vi "main.vi"() -> ()   [LabVIEW 2014]
uses:
  typedef/ctlPlot.ctl
  typedef/ePMUConfig.ctl
  typedef/eStepType.ctl
  typedef/eStepDir.ctl
  typedef/rdoTestType.ctl
  typedef/appState.ctl
  typedef/eRptType.ctl
  typedef/PMUConfig.ctl
panel:
  out "Uncertainties":dbl[][][](array[numeric]) format="%#_2g"
  in  "rdoTest Type":T1
  in  "btnSave":bool
  in  "btnCalcPFI":bool
  in  "btnCalcRT":bool
  in  "DONE":bool
  in  "Tab Control":T2(tab)
  in  "UncertPage":enum16{"50 Hz", "60 Hz"}(ring) caption="Nominal Freq"
  out "Uncert Table":string[][](table)
  out "StepLimits":dbl[][][](array[numeric]) caption="Step Test Limits" format="%#_4f"
  in  "Limit Page":T3 caption="PMU Config"
  out "Limits":dbl[][][](array[numeric]) caption="TVE, FE, RFE Limits"
  in  "btnSaveTUR":bool
  out "TUR":dbl[][][](array[numeric])
  in  "TUR Page":T3 caption="PMU Config"
  in  "full_temp_PFI":enum32{"full", "temp"}(tab)
  in  "PFI Page":T3 caption="PMU Config"
  out "PFI":string[][][](array[string])
  out "Temp Test PFI":string[][][](array[string])
  in  "TempFreq":enum16{"50 Hz", "60 Hz"}(ring) caption="Nominal Freq"
  out "RTPFI":string[][][](array[string]) caption="Pass/Fail/Indeterminate"
  in  "eRTDir":T4 caption="Step Direction"
  in  "eRTType":T5 caption="Step Type"
  out "RTUncert":dbl[][][][][](array[numeric]) caption="Resp Time Uncert"
  out "RTRange":dbl[][][][][](array[numeric]) caption="Resp Time Range"
  in  "eRTPage":T3 caption="PMU Config"
  out "DlyTimePFI":string[][][](array[string])
  in  "eDTDir":T4 caption="Step Direction"
  in  "eDTType":T5 caption="Step Type"
  in  "eDTPage":T3 caption="PMU Config"
  out "DlyTimeRng":dbl[][][][][](array[numeric]) format="%.6f"
  in  "eOvrDir":T4 caption="Step Direction"
  in  "eOvrType":T5 caption="Step Type"
  in  "eOvrUndrPage":T3 caption="PMU Config"
  out "OvrUndrPFI":string[][][][][](array[string])
  out "OvrUndr":dbl[][][][][](array[numeric])=[[[[[5.598492295160192, 5.589160017980474, 5.579827740800756, 6.2090278478135055, 6.202935187769419, 6.196842527725332, 6.270368754436869, 6.261733208094874, 6.2530976617528795, 5.499241138114173, 5.4912209769255735, 5.483200815736974, 5.591363005137677, 5.589161707344972, 5.586960409552266, 6.2034021327898525, 6.2029551231392706, 6.202508113488689, 6.262186470202315, 6.261747037530138, 6.261307604857961, 5.492149609028501, 5.491120362323346, 5.490091115618191], [4.582281382800085, 4.572949105620367, 4.563616828440649, 2.0737377226338936, 2.0676450625898064, 2.0615524025457193, 1.1136472889469742, 1.1050117426049793, 1.0963761962629843, 4.500837324127726, 4.492817162939127, 4.484797001750527, 4.57515178562041, 4.572950487827704, 4.570749190034999, 2.068098717363672, 2.06765170771309, 2.067204698062508, 1.1054536157657309, 1.1050141830935536, 1.1045747504213763, 4.493764088606066, 4.492734841900911, 4.491705595195756], [6.26023399342542, 6.250901716245702, 6.241569439065984, 6.128438171518977, 6.12234551147489, 6.116252851430803, 6.430675694174775, 6.422040147832781, 6.413404601490786, 6.102855597590311, 6.094835436401712, 6.086815275213112, 6.253149166340811, 6.2509478685481055, 6.2487465707554, 6.122858708702316, 6.122411699051734, 6.121964689401152, 6.422526817417168, 6.422087384744991, 6.421647952072814, 6.095816462969536, 6.094787216264381, 6.093757969559226], [3.375202432081235, 3.3658701549015175, 3.3565378777218, 3.302740243145951, 3.296647583101864, 3.2905549230577766, 1.1419367489007164, 1.1333012025587215, 1.1246656562167265, 2.0396319733224955, 2.0316118121338955, 2.0235916509452956, 3.368096303933992, 3.3658950061412862, 3.3636937083485803, 3.297130232216894, 3.296683222566312, 3.29623621291573, 1.1337489711565862, 1.133309538484409, 1.1328701058122317, 2.0326249854599556, 2.0315957387548007, 2.030566492049646]], [[5.6114389386325305, 5.602495822485004, 5.593552706337477, 6.4971644746473425, 6.4906779148884395, 6.4841913551295365, 6.452789687138199, 6.442635198982573, 6.432480710826947, 5.499700075652654, 5.491172020965302, 5.4826439662779505, 5.604365790119637, 5.602470106718821, 5.600574423318005, 6.491501742716185, 6.490751963178685, 6.4900021836411845, 6.443115798655941, 6.442548550239463, 6.4419813018229855, 5.492187667629821, 5.4911167638448894, 5.490045860059958], [4.592803334544344, 4.583860218396818, 4.574917102249291, 1.1519003094451032, 1.1454137496861998, 1.1389271899272964, 2.1576995544831505, 2.147545066327524, 2.1373905781718974, 4.501305162749851, 4.4927771080625, 4.484249053375148, 4.585734861625306, 4.58383917822449, 4.5819434948236735, 1.146176596569033, 1.1454268170315325, 1.144677037494032, 2.148083431829625, 2.1475161834131473, 2.1469489349966695, 4.4938028014762015, 4.49273189769127, 4.491660993906338], [5.824200079831354, 5.815256963683828, 5.806313847536301, 6.213851725577966, 6.207365165819063, 6.20087860606016, 6.175131282852548, 6.164976794696922, 6.154822306541296, 6.103387438698514, 6.094859384011162, 6.08633132932381, 5.81714404673894, 5.815248363338124, 5.813352679937307, 6.208174990295637, 6.207425210758137, 6.206675431220637, 6.165428416601619, 6.1648611681851415, 6.164293919768664, 6.095893577165425, 6.094822673380493, 6.093751769595562], [3.140235327361881, 3.1312922112143546, 3.1223490950668285, 1.101903941962272, 1.0954173822033686, 1.0889308224444652, 2.0651467530546004, 2.054992264898974, 2.044837776743347, 2.040147849357748, 2.0316197946703958, 2.0230917399830437, 3.133183263659809, 3.131287580258993, 3.1293918968581766, 1.0961777579065755, 1.095427978369075, 1.0946781988315746, 2.0555209711448583, 2.0549537227283805, 2.0543864743119027, 2.032678461578429, 2.0316075577934978, 2.0305366540085665]]]]] caption="Overshoot in Percent (%)" format="%.2f"
  out "StepPlot":cluster{"Array":dbl[], "Array":dbl[]}(graph)
  in  "ctlPlot":T6
  out "Step TVE":cluster{"Array":dbl[], "Array":dbl[]}(graph)
  in  "ePlotPage":T3 caption="PMU Config"
  in  "ePlotType":enum16{"Phase", "Magnitude"}(ring) caption="Step Type"
  in  "ePlotDir":enum16{"Pos", "Neg"}(ring) caption="Step Direction"
  out "error out":errorcluster
  in  "error in (no error)":errorcluster
  # "VC"
  # "IA"
  # "VB"
  # "V+"
  # "IB"
  # "IC"
  # "I+"
  # "FREQ"
  # "ROCOF"
  # "VA"
  # "Step Resp Time (s)"
  # "Step Delay Time (s)"
  # "Step Ovr/Undr  (%)"
  # "VA TVE"
  # "VB TVE"
  # "VC TVE"
  # "V+ TVE"
  # "IA TVE"
  # "IB TVE"
  # "IC TVE"
  # "I+ TVE"
  # "FE"
  # "RFE"
  # "FreqRng"
  # "MagRng"
  # "Harm"
  # "OOB"
  # "Phase Mod"
  # "Ampl Mod"
  # "Ramp +"
  # "Ramp -"
  # "VA"
  # "VB"
  # "VC"
  # "V+"
  # "IA"
  # "IB"
  # "IC"
  # "I+"
  # "FREQ"
  # "ROCOF"
  # "FreqRng"
  # "MagRng"
  # "Harm"
  # "OOB"
  # "Phase Mod"
  # "Ampl Mod"
  # "Ramp +"
  # "Ramp -"
  # "VA TVE"
  # "VB TVE"
  # "VC TVE"
  # "V+ TVE"
  # "IA TVE"
  # "IB TVE"
  # "IC TVE"
  # "I+ TVE"
  # "FE"
  # "RFE"
  # "FreqRng"
  # "MagRng"
  # "Harm"
  # "OOB"
  # "Phase Mod"
  # "Ampl Mod"
  # "Freq Ramp +"
  # "Freq Ramp -"
  # "60F0_10Fs_M_50C\n\n60F0_10Fs_M_50C\n\n60F0_10Fs_P_50C\n\n60F0_10Fs_P_0C\n\n60F0_12Fs_M_50C\n\n60F0_12Fs_M_0C\n\n60F0_12Fs_P_50C\n\n60F0_12Fs_P_0C\n\n60F0_15Fs_M_50C\n\n60F0_15Fs_M_0C\n\n60F0_15Fs_P_50C\n\n60F0_15Fs_P_0C\n\n60F0_20Fs_M_50C\n\n60F0_20Fs_M_0C\n\n60F0_20Fs_P_50C\n\n60F0_20Fs_P_0C\n\n60F0_30Fs_M_50C\n\n60F0_30Fs_M_0C\n60F0_30Fs_P_50C\n\n60F0_30Fs_P_0C\n\n60F0_60Fs_M_50C\n\n60F0_60Fs_M_0C\n\n60F0_60Fs_P_50C\n\n60F0_60Fs_P_0C"
  # "50F0_10Fs_M_50C\n\n50F0_10Fs_M_0C\n\n50F0_10F0_P_50C\n\n50F0_10Fs_P_0C\n\n50F0_25Fs_M_50C\n\n50F0_25Fs_M_0C\n\n50F0_25Fs_P_50C\n\n50F0_25Fs_P_0C\n\n50F0_50Fs_M_50C\n\n50F0_50Fs_M_0C\n\n50F0_50Fs_P_50C\n\n50F0_50Fs_P_0C"
  # "VA TVE"
  # "VB TVE"
  # "VC TVE"
  # "V+ TVE"
  # "IA TVE"
  # "IB TVE"
  # "IC TVE"
  # "I+ TVE"
  # "FE"
  # "RFE"
  # "VA                      VB                     VC                     V+                     IA                         IB                    IC                            I+                  Freq                    ROCOF"
  # "Phase Step Positive RT"
  # "Phase Step Negative RT"
  # "Magnitude Step Positive RT"
  # "Magnitude Step Positive RT"
  # "VA                      VB                     VC                     V+                     IA                         IB                    IC                            I+                  Freq                    ROCOF"
  # "plus\n\nRT\n\nminus"
  # "VA                      VB                     VC                     V+                     IA                         IB                    IC                            I+                  Freq                    ROCOF"
  # "RT + unc\n\nRT\n\nRT - unc"
  # "VA"
  # "VB"
  # "VC"
  # "V+"
  # "IA"
  # "IB"
  # "IC"
  # "I+"
  # "Phase Step Pos"
  # "Phase Step Neg"
  # "Mag Step Pos"
  # "Mag Step Neg"
  # "VA"
  # "VB"
  # "VC"
  # "V+"
  # "IA"
  # "IB"
  # "IC"
  # "I+"
  # "DT + Unc"
  # "DT"
  # "DT - Unc"
  # "VA"
  # "VB"
  # "VC"
  # "V+"
  # "IA"
  # "IB"
  # "IC"
  # "I+"
  # "PreOvr"
  # "PreUndr"
  # "PostOvr"
  # "PostUndr"
  # "VA+u"
  # "VA"
  # "VA-u"
  # "VB+u"
  # "VB"
  # "VB-u"
  # "VC+u"
  # "VCB"
  # "VC-u"
  # "V+u"
  # "V+B"
  # "V+-u"
  # "IA+u"
  # "IA"
  # "IA-u"
  # "IB+u"
  # "IB"
  # "IB-u"
  # "IC+u"
  # "IC"
  # "IC-u"
  # "I++u"
  # "I+B"
  # "I+-u"
  # "PreOvr"
  # "PreUndr"
  # "PostOvr"
  # "PostUndr"
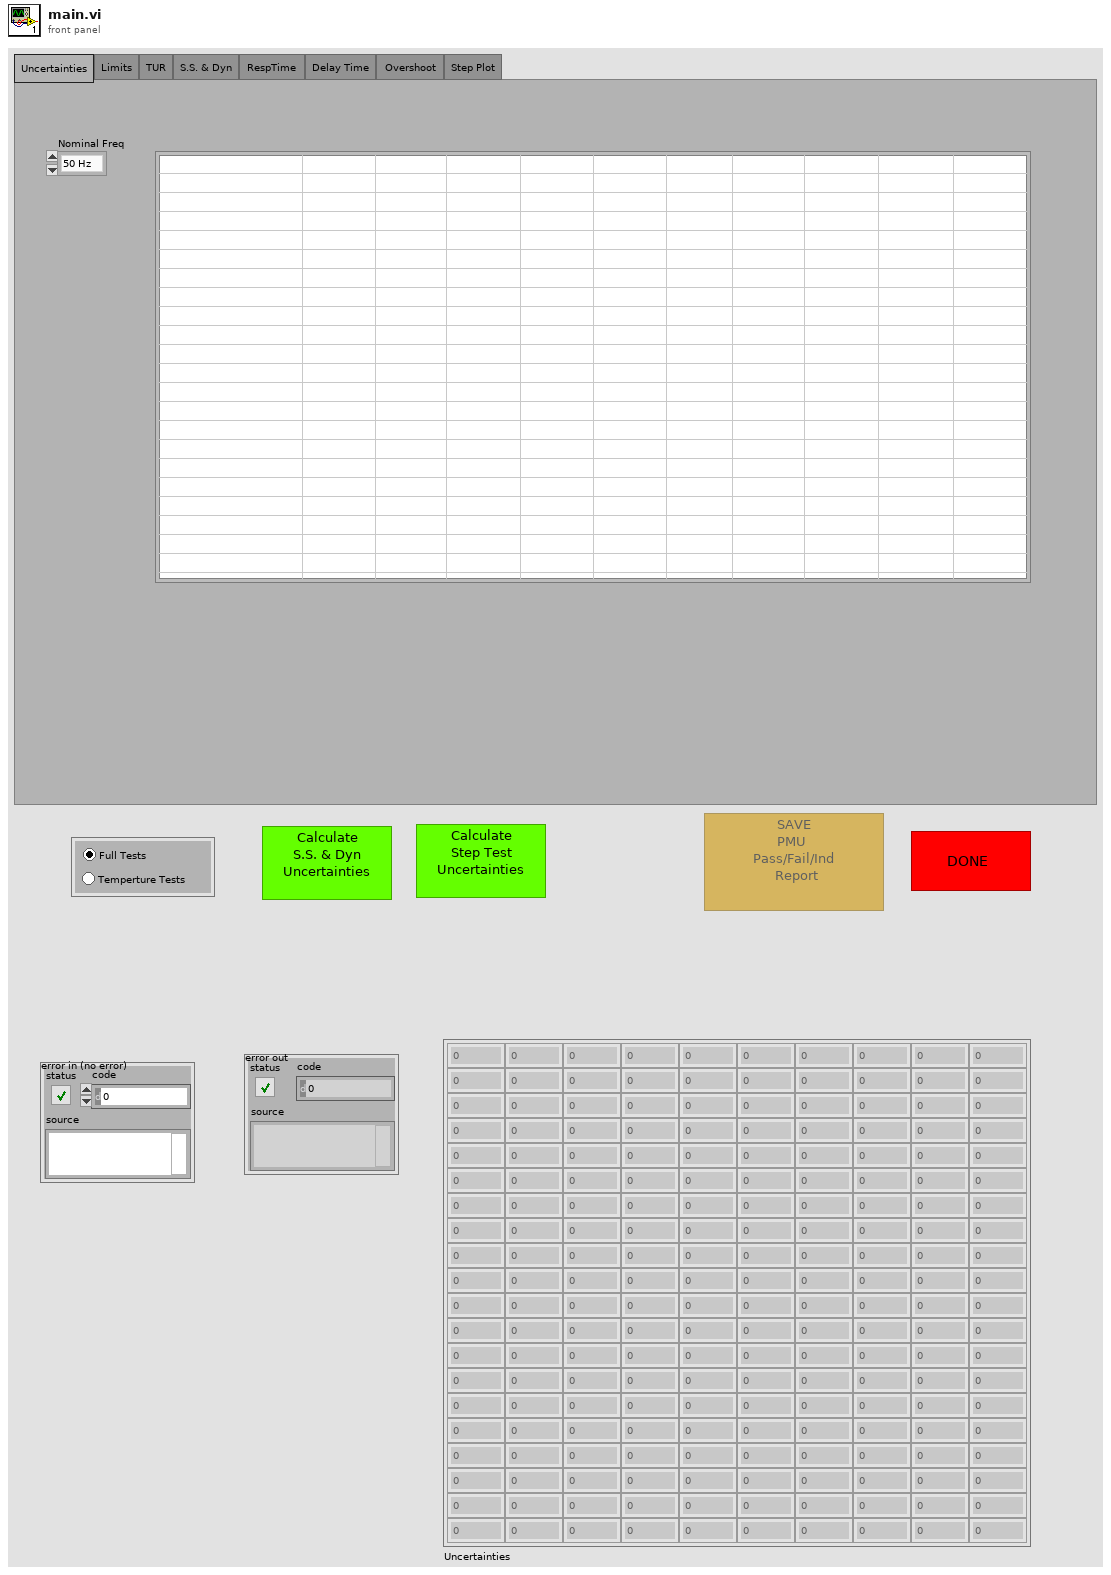
[diagram p1: front panel]
types:
  T1 = typedef "rdoTestType.ctl" = enum32{"rFull", "rTemp"}
  T2 = enum32{"Uncertainties", "Limits", "TUR", "S.S. & Dyn", "RespTime ", "Delay Time", "Overshoot ", "Step Plot"}
  T3 = typedef "ePMUConfig.ctl" = enum16{"50F0 10Fs M", "50F0 10Fs P", "50F0 25Fs M", "50F0 25Fs P", "50F0 50Fs M", "50F0 50Fs P", "60F0 10Fs M", "60F0 10Fs P", "60F0 12Fs M", "60F0 12Fs P", "60F0 15Fs M", "60F0 15Fs P", "60F0 20Fs M", "60F0 20Fs P", "60F0 30Fs M", "60F0 30Fs P", "60F0 60Fs M", "60F0 60Fs P"}
  T4 = typedef "eStepDir.ctl" = enum16{"Pos", "Neg"}
  T5 = typedef "eStepType.ctl" = enum16{"Phase", "Magnitude"}
  T6 = typedef "ctlPlot.ctl" = cluster{"Channel":enum16{"VA", "VB", "VC", "V+", "IA", "IB", "IC", "I+", "FREQ", "ROCOF"}, "Parameter":enum16{"TVE", "ME", "PE"}}
  T7 = enum8{"Enabled", "Disabled", "Disabled and Grayed Out"}
  T8 = typedef "appState.ctl" = enum16{"init", "processUI", "exit"}
  T9 = typedef "eRptType.ctl" = enum16{"get", "Clear", "Set Temp", "Set PFI", "Set Step"}
  T10 = typedef "PMUConfig.ctl" = cluster{"Class":string, "Fs":dbl, "F0":dbl}
  T11 = enum16{"get", "Clear", "Set Temp", "Set PFI", "Set Step"}
  T12 = cluster{"DlyTimeRng":dbl[][][][][], "DlyTimePFI":string[][][]}
  T13 = cluster{"OvrUndr":dbl[][][][][], "OvrUndrPFI":string[][][][][]}
  T14 = cluster{"RT Range":dbl[][][][][], "RT Uncert":dbl[][][][][], "RT_PFI":string[][][]}
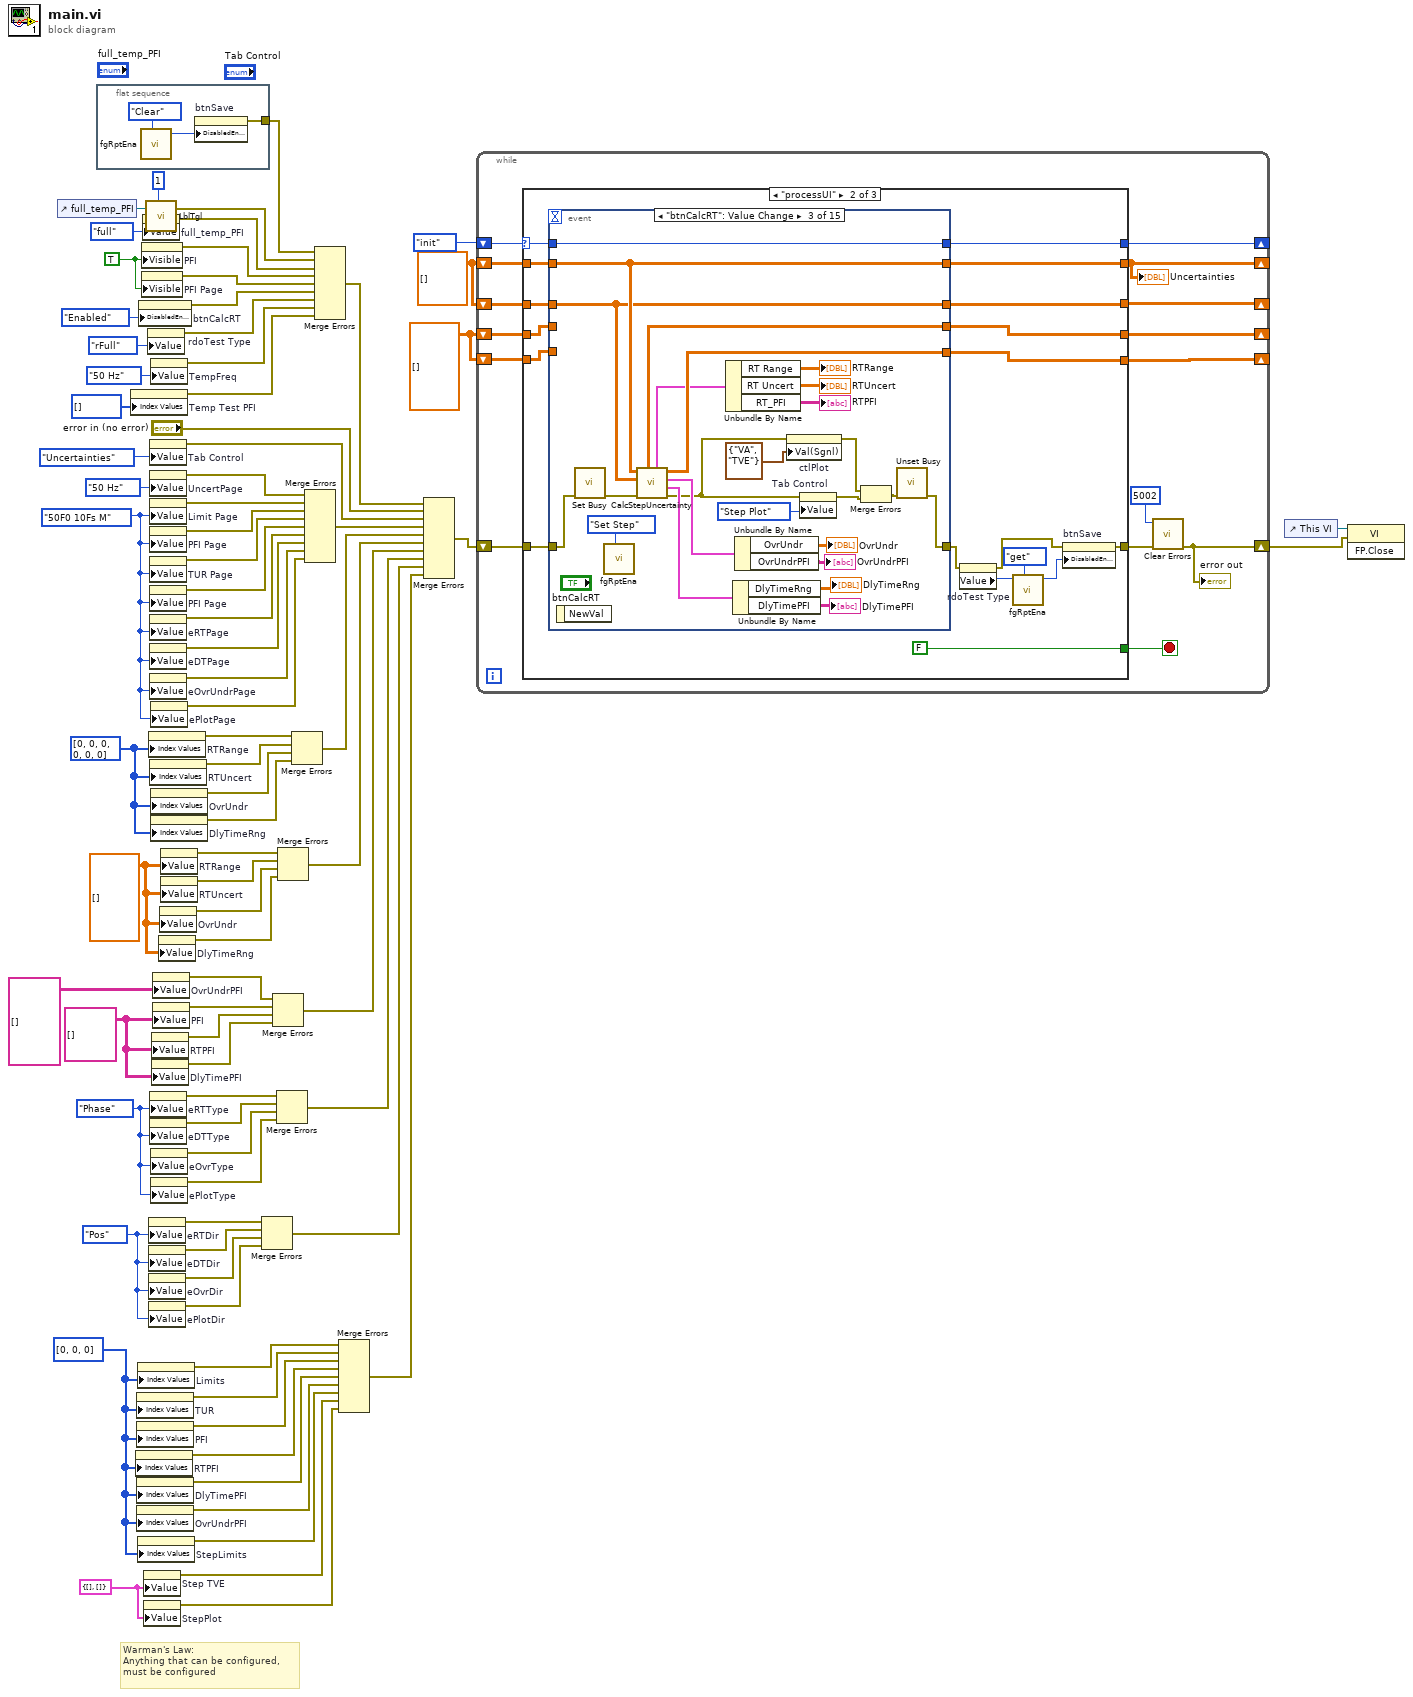
[diagram p0: block diagram]
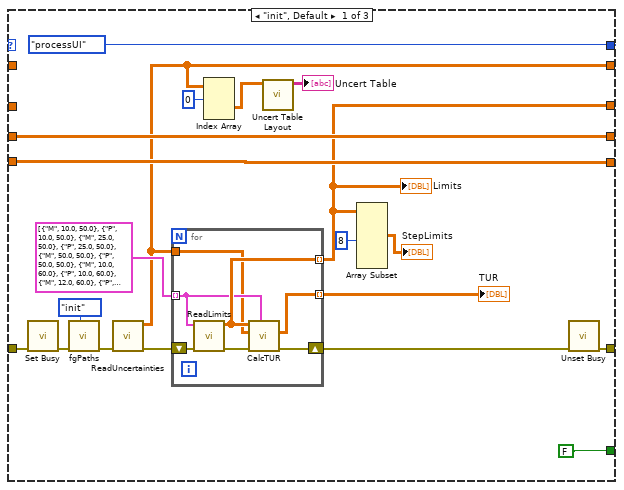
[diagram p2: hidden frame]
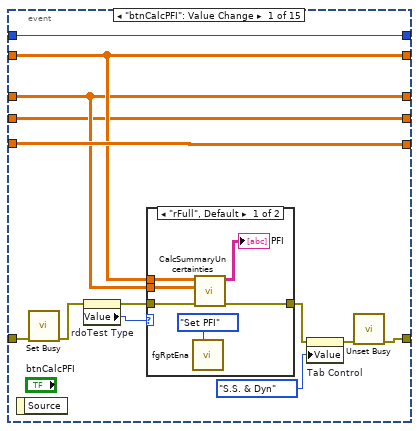
[diagram p3: hidden frame]
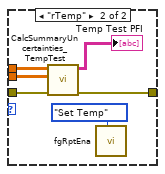
[diagram p4: hidden frame]
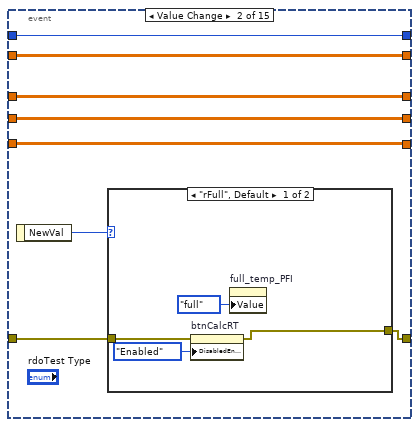
[diagram p5: hidden frame]
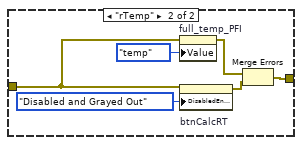
[diagram p6: hidden frame]
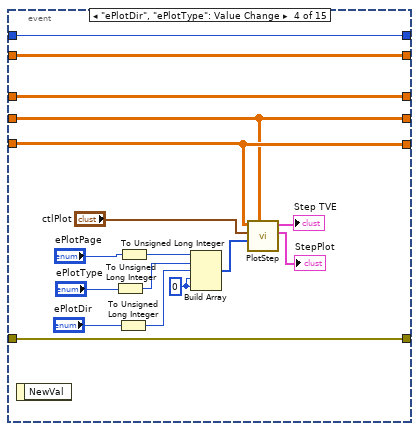
[diagram p7: hidden frame]
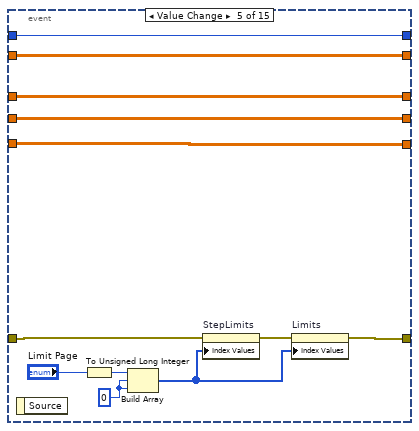
[diagram p8: hidden frame]
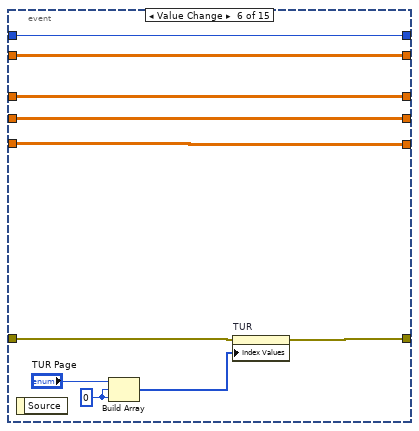
[diagram p9: hidden frame]
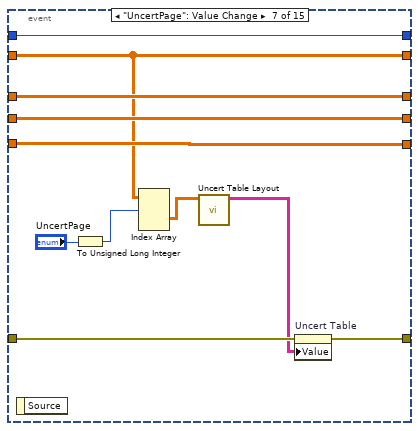
[diagram p10: hidden frame]
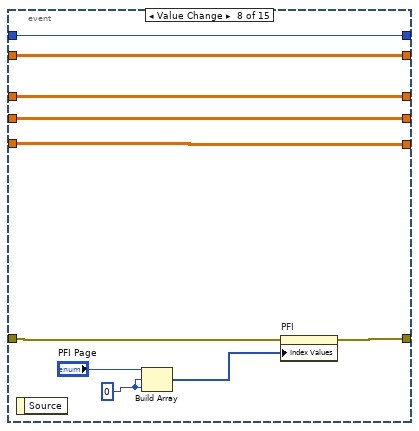
[diagram p11: hidden frame]
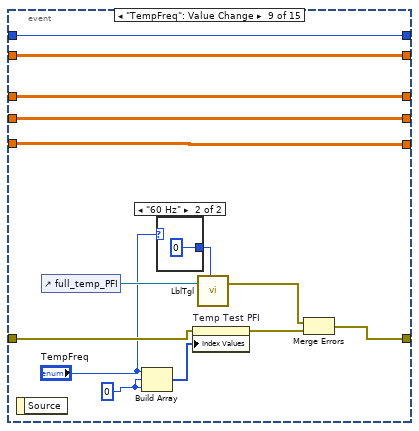
[diagram p12: hidden frame]
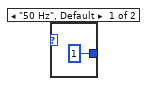
[diagram p13: hidden frame]
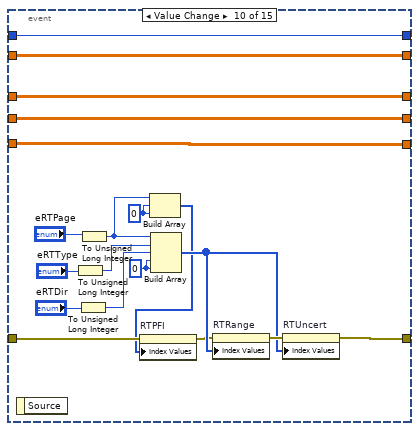
[diagram p14: hidden frame]
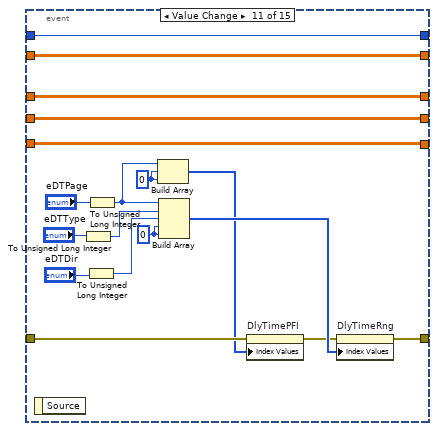
[diagram p15: hidden frame]
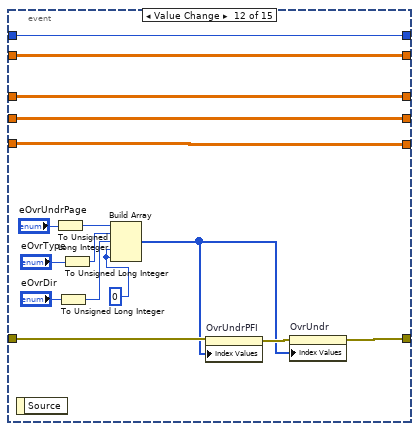
[diagram p16: hidden frame]
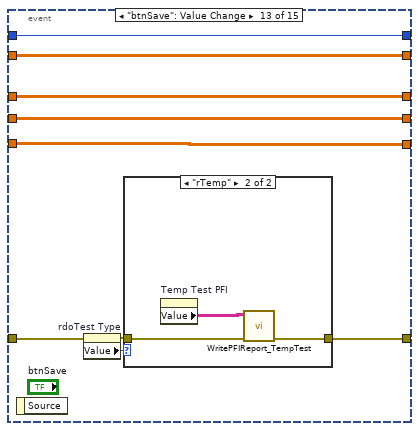
[diagram p17: hidden frame]
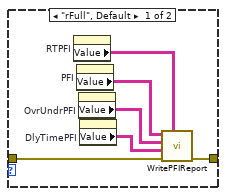
[diagram p18: hidden frame]
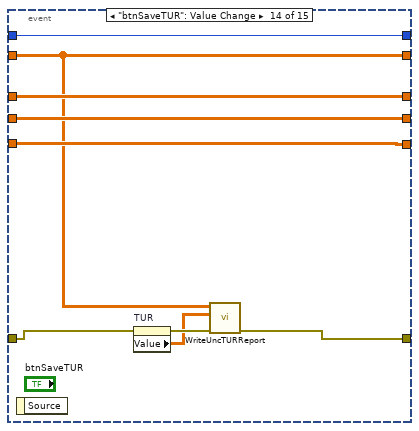
[diagram p19: hidden frame]
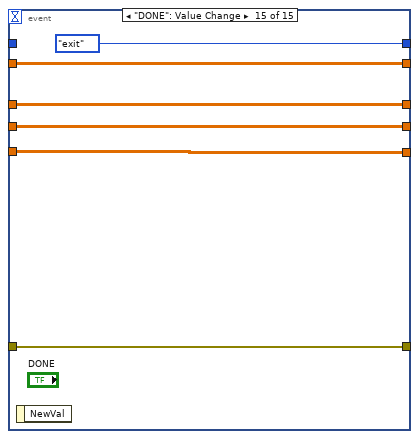
[diagram p20: hidden frame]
diagram:
  w10 = TRUE ("Visible")
  w21 = cluster{"Array":dbl[], "Array":dbl[]} {"Array"=[], "Array"=[]} ("Step TVE")
  w43 = eStepDir."Pos" ("eRTDir")
  w48 = eStepType."Phase" ("eRTType")
  w59 = u32[] [0, 0, 0, 0, 0, 0] ("Index Values")
  w30 = string[][][] [] ("PFI")
  w71 = dbl[][][][][] [] ("Range")
  w50 = ePMUConfig."50F0 10Fs M" ("Limit Page")
  w23 = u32[] [0, 0, 0] ("Index Values")
  w74 = dbl[][][][][] [] ("Step Data")
  w78 = dbl[][][] []
  # "Warman's Law:\nAnything that can be configured,\nmust be configured"
  n1 = control-ref of="full_temp_PFI"() -> (w82:refnum<vi>)
  n2 = flat-sequence {
    tunnel: [w84] -> w2
    frame #0 {
      n3 = call "fgRptEna.vi"("eRptType"=eRptType."Clear" ("Enum")) -> ("ENA"=w83:T7)  [unwired: 10 in]
      n4 = property on="btnSave" class="Bool"("DisabledEnum"=w83) -> (error out=w84:errorcluster)  [unwired: 2 in, 1 out]
    }
  }
  n5 = property on="Temp Test PFI" class="Arr (strict)"("Index Values"=u32[] []) -> (error out=w3:errorcluster)  [unwired: 2 in, 1 out]
  n6 = property on="RTPFI" class="Arr (strict)"("Index Values"=w23) -> (error out=w66:errorcluster)  [unwired: 2 in, 1 out]
  n7 = property on="TUR" class="Arr (strict)"("Index Values"=w23) -> (error out=w68:errorcluster)  [unwired: 2 in, 1 out]
  n8 = property on="PFI" class="Arr (strict)"("Index Values"=w23) -> (error out=w67:errorcluster)  [unwired: 2 in, 1 out]
  n9 = property on="DlyTimePFI" class="Arr (strict)"("Index Values"=w23) -> (error out=w65:errorcluster)  [unwired: 2 in, 1 out]
  n10 = property on="OvrUndrPFI" class="Arr (strict)"("Index Values"=w23) -> (error out=w64:errorcluster)  [unwired: 2 in, 1 out]
  n11 = property on="Limits" class="Arr (strict)"("Index Values"=w23) -> (error out=w69:errorcluster)  [unwired: 2 in, 1 out]
  n12 = property on="StepLimits" class="Arr (strict)"("Index Values"=w23) -> (error out=w22:errorcluster)  [unwired: 2 in, 1 out]
  n13 = property on="btnCalcRT" class="Bool"("DisabledEnum"=T7."Enabled" ("Disabled")) -> (error out=w12:errorcluster)  [unwired: 2 in, 1 out]
  n14 = property on="PFI" class="Arr (strict)"("Visible"=w10) -> (error out=w14:errorcluster)  [unwired: 2 in, 1 out]
  n15 = property on="PFI Page" class="Enum (strict)"("Visible"=w10) -> (error out=w15:errorcluster)  [unwired: 2 in, 1 out]
  n16 = property on="full_temp_PFI" class="TabCtl (strict)"("Value"=enum32{"full", "temp"}."full" ("full_temp_PFI")) -> (error out=w8:errorcluster)  [unwired: 2 in, 1 out]
  n17 = property on="Step TVE" class="XYGraph (strict)"("Value"=w21) -> (error out=w20:errorcluster)  [unwired: 2 in, 1 out]
  n18 = property on="StepPlot" class="XYGraph (strict)"("Value"=w21) -> (error out=w19:errorcluster)  [unwired: 2 in, 1 out]
  n19 = call "LblTgl.vi"("TabControl in"=w82, "Numeric"=1) -> ("error out"=w7:errorcluster)  [unwired: 17 in]
  n20 = property on="rdoTest Type" class="RadioBtnsControl (strict)"("Value"=enum32{"rFull", "rTemp"}."rFull" ("Test Type")) -> (error out=w11:errorcluster)  [unwired: 2 in, 1 out]
  n21 = property on="RTRange" class="Arr (strict)"("Index Values"=w59) -> (error out=w63:errorcluster)  [unwired: 2 in, 1 out]
  n22 = property on="eRTDir" class="Enum (strict)"("Value"=w43) -> (error out=w42:errorcluster)  [unwired: 2 in, 1 out]
  n23 = property on="eDTDir" class="Enum (strict)"("Value"=w43) -> (error out=w41:errorcluster)  [unwired: 2 in, 1 out]
  n24 = property on="eOvrDir" class="Enum (strict)"("Value"=w43) -> (error out=w40:errorcluster)  [unwired: 2 in, 1 out]
  n25 = property on="ePlotDir" class="Enum (strict)"("Value"=w43) -> (error out=w39:errorcluster)  [unwired: 2 in, 1 out]
  n26 = property on="Tab Control" class="TabCtl (strict)"("Value"=T2."Uncertainties" ("Tab Control")) -> (error out=w25:errorcluster)  [unwired: 2 in, 1 out]
  n27 = property on="UncertPage" class="Enum (strict)"("Value"=enum16{"50 Hz", "60 Hz"}."50 Hz" ("UncertPage")) -> (error out=w51:errorcluster)  [unwired: 2 in, 1 out]
  n28 = property on="Limit Page" class="Enum (strict)"("Value"=w50) -> (error out=w58:errorcluster)  [unwired: 2 in, 1 out]
  n29 = property on="PFI Page" class="Enum (strict)"("Value"=w50) -> (error out=w57:errorcluster)  [unwired: 2 in, 1 out]
  n30 = property on="TUR Page" class="Enum (strict)"("Value"=w50) -> (error out=w56:errorcluster)  [unwired: 2 in, 1 out]
  n31 = property on="PFI Page" class="Enum (strict)"("Value"=w50) -> (error out=w55:errorcluster)  [unwired: 2 in, 1 out]
  n32 = property on="eRTPage" class="Enum (strict)"("Value"=w50) -> (error out=w54:errorcluster)  [unwired: 2 in, 1 out]
  n33 = property on="eDTPage" class="Enum (strict)"("Value"=w50) -> (error out=w53:errorcluster)  [unwired: 2 in, 1 out]
  n34 = property on="eOvrUndrPage" class="Enum (strict)"("Value"=w50) -> (error out=w52:errorcluster)  [unwired: 2 in, 1 out]
  n35 = property on="RTUncert" class="Arr (strict)"("Index Values"=w59) -> (error out=w62:errorcluster)  [unwired: 2 in, 1 out]
  n36 = property on="eRTType" class="Enum (strict)"("Value"=w48) -> (error out=w47:errorcluster)  [unwired: 2 in, 1 out]
  n37 = property on="eDTType" class="Enum (strict)"("Value"=w48) -> (error out=w46:errorcluster)  [unwired: 2 in, 1 out]
  n38 = property on="TempFreq" class="Enum (strict)"("Value"=enum16{"50 Hz", "60 Hz"}."50 Hz" ("TempFreq")) -> (error out=w5:errorcluster)  [unwired: 2 in, 1 out]
  n39 = property on="ePlotPage" class="Enum (strict)"("Value"=w50) -> (error out=w49:errorcluster)  [unwired: 2 in, 1 out]
  n40 = property on="OvrUndr" class="Arr (strict)"("Index Values"=w59) -> (error out=w61:errorcluster)  [unwired: 2 in, 1 out]
  n41 = property on="DlyTimeRng" class="Arr (strict)"("Index Values"=w59) -> (error out=w60:errorcluster)  [unwired: 2 in, 1 out]
  n42 = property on="eOvrType" class="Enum (strict)"("Value"=w48) -> (error out=w45:errorcluster)  [unwired: 2 in, 1 out]
  n43 = property on="ePlotType" class="Enum (strict)"("Value"=w48) -> (error out=w44:errorcluster)  [unwired: 2 in, 1 out]
  n44 = property on="RTPFI" class="Arr (strict)"("Value"=w30) -> (error out=w72:errorcluster)  [unwired: 2 in, 1 out]
  n45 = property on="DlyTimePFI" class="Arr (strict)"("Value"=w30) -> (error out=w28:errorcluster)  [unwired: 2 in, 1 out]
  n46 = property on="OvrUndrPFI" class="Arr (strict)"("Value"=string[][][][][] [] ("OvrUndrPFI")) -> (error out=w27:errorcluster)  [unwired: 2 in, 1 out]
  n47 = property on="PFI" class="Arr (strict)"("Value"=w30) -> (error out=w73:errorcluster)  [unwired: 2 in, 1 out]
  n48 = property on="DlyTimeRng" class="Arr (strict)"("Value"=w71) -> (error out=w70:errorcluster)  [unwired: 2 in, 1 out]
  n49 = property on="OvrUndr" class="Arr (strict)"("Value"=w71) -> (error out=w75:errorcluster)  [unwired: 2 in, 1 out]
  n50 = property on="RTRange" class="Arr (strict)"("Value"=w71) -> (error out=w77:errorcluster)  [unwired: 2 in, 1 out]
  n51 = property on="RTUncert" class="Arr (strict)"("Value"=w71) -> (error out=w76:errorcluster)  [unwired: 2 in, 1 out]
  n52 = Merge Errors(w42, w41, w40, w39) -> (w33:errorcluster)
  n53 = Merge Errors(w27, w73, w72, w28) -> (w35:errorcluster)
  n54 = Merge Errors(w47, w46, w45, w44) -> (w34:errorcluster)
  n55 = Merge Errors(w77, w76, w75, w70) -> (w36:errorcluster)
  n56 = Merge Errors(w63, w62, w61, w60) -> (w37:errorcluster)
  n57 = Merge Errors(w51, w58, w57, w56, w55, w54, w53, w52, w49) -> (w38:errorcluster)
  n58 = Merge Errors(w2, w7, w8, w14, w15, w12, w11, w5, w3) -> (w13:errorcluster)
  n59 = Merge Errors(w69, w68, w67, w66, w65, w64, w22, w20, w19) -> (w32:errorcluster)
  n60 = Merge Errors(w13, "error in (no error)", w25, w38, w37, w36, w35, w34, w33, w32) -> (w31:errorcluster)
  n61 = while {
    shift-right: [w98] -> _
    shift-left: appState."init" ("AppState") -> [w100]
    shift-right: [w90] -> w18
    shift-left: w31 -> [w97]
    shift-right: [w95] -> _
    shift-left: w78 -> [w96]
    shift-right: [w93] -> _
    shift-left: w74 -> [w94]
    shift-right: [w91] -> _
    shift-left: w78 -> [w92]
    shift-right: [w86] -> _
    shift-left: w74 -> [w87]
    stop <- w99 stop-if-true
    n62 = case shown="\"processUI\"" w100 {
      selector: w100 -> [_ w138 _]
      tunnel: [FALSE FALSE TRUE] -> w99
      tunnel: [appState."processUI" ("AppState") w143 appState."exit" ("AppState")] -> w98
      tunnel: [w110 w133 w379] -> w89
      tunnel: w97 -> [w112 w144 w379]
      tunnel: [w104 w142 w380] -> w95
      tunnel: w96 -> [_ w141 w380]
      tunnel: [w118 w140 w378] -> w93
      tunnel: w94 -> [w118 w139 w378]
      tunnel: w92 -> [_ w137 w377]
      tunnel: [w108 w136 w377] -> w91
      tunnel: w87 -> [w109 w135 w376]
      tunnel: [w109 w134 w376] -> w86
      frame "init", Default {
        n63 = call <vilib>:"Set Busy.vi"("error in (no error)"=w112) -> ("error out"=w111:errorcluster)  [unwired: 9 in, 1 out]
        n64 = call "fgPaths.vi"("cmd"=enum16{"init", "set", "get"}."init", "error in (no error)"=w111) -> ("error out"=w114:errorcluster)  [unwired: 8 in, 1 out]
        n65 = call "ReadUncertainties.vi"("error in (no error)"=w114) -> ("error out"=w117:errorcluster, "Uncertainties"=w104:dbl[][][])  [unwired: 8 in]
        n66 = for {
          shift-right: [w125] -> w105
          shift-left: w117 -> [w127]
          tunnel: T10[] [{"Class"="M", "Fs"=10.0, "F0"=50.0}, {"Class"="P", "Fs"=10.0, "F0"=50.0}, {"Class"="M", "Fs"=25.0, "F0"=50.0}, {"Class"="P", "Fs"=25.0, "F0"=50.0}, {"Class"="M", "Fs"=50.0, "F0"=50.0}, {"Class"="P", "Fs"=50.0, "F0"=50.0}, {"Class"="M", "Fs"=10.0, "F0"=60.0}, {"Class"="P", "Fs"=10.0, "F0"=60.0}, {"Class"="M", "Fs"=12.0, "F0"=60.0}, {"Class"="P", "Fs"=12.0, "F0"=60.0}, {"Class"="M", "Fs"=15.0, "F0"=60.0}, {"Class"="P", "Fs"=15.0, "F0"=60.0}, {"Class"="M", "Fs"=20.0, "F0"=60.0}, {"Class"="P", "Fs"=20.0, "F0"=60.0}, {"Class"="M", "Fs"=30.0, "F0"=60.0}, {"Class"="P", "Fs"=30.0, "F0"=60.0}, {"Class"="M", "Fs"=60.0, "F0"=60.0}, {"Class"="P", "Fs"=60.0, "F0"=60.0}] -> [w123] mode=indexing
          tunnel: [w124] -> w108 mode=indexing
          tunnel: w104 -> [w122]
          tunnel: [w121] -> w115 mode=indexing
          n67 = call "ReadLimits.vi"("error in (no error)"=w127, "PMUConfig"=w123) -> ("error out"=w126:errorcluster, "Limits"=w124:dbl[][])  [unwired: 8 in]
          n68 = call "CalcTUR.vi"("PMUConfig"=w123, "error in (no error)"=w126, "Uncertainties"=w122, "Limits"=w124) -> ("error out"=w125:errorcluster, "TUR"=w121:dbl[][])  [unwired: 6 in]
        }
        "TUR" <- w115
        "Limits" <- w108
        n69 = Index Array(array=w104, index (dim 0)=0 ("index (page)")) -> (element=w102:dbl[][])  [unwired: 2 in]
        n70 = call "Uncert Table Layout.vi"("Uncert In"=w102) -> ("Uncert Table"=→"Uncert Table":string[][])  [unwired: 10 in]
        n71 = Array Subset(array=w108, index (dim 1)=8 ("index")) -> (→"StepLimits":dbl[][][])  [unwired: 5 in]
        n72 = call <vilib>:"Unset Busy.vi"("error in (no error)"=w105) -> ("error out"=w110:errorcluster)  [unwired: 10 in]
      }
      frame "processUI" {
        n73 = event shown="[2] \"btnCalcRT\": Value Change" {
          selector: _ -> [_ _ _ _ _ _ _ _ _ _ _ _ _ _ _]
          dyn-events: _ -> [_ _ _ _ _ _ _ _ _ _ _ _ _ _ _]
          timeout: _ -> [_ _ _ _ _ _ _ _ _ _ _ _ _ _ _]
          tunnel: [w153 w171 w207 w227 w239 w252 w254 w273 w277 w304 w313 w333 w347 w365 w375] -> w131
          tunnel: w144 -> [w154 w172 w209 w227 w233 w247 w255 w272 w279 w293 w310 w335 w344 w364 w375]
          tunnel: [w156 w177 w213 w230 w238 w251 w262 w268 w286 w308 w326 w342 w351 w369 appState."exit" ("AppState")] -> w143
          tunnel: [w157 w178 w212 w229 w237 w250 w258 w267 w285 w307 w325 w341 w350 w361 w373] -> w142
          tunnel: w141 -> [w157 w178 w212 w229 w237 w250 w258 w267 w285 w307 w325 w341 w350 w361 w373]
          tunnel: [w158 w174 w210 w221 w235 w248 w260 w265 w283 w305 w322 w339 w348 w366 w372] -> w140
          tunnel: w139 -> [w158 w174 _ w221 w235 w248 w260 w265 w283 w305 w322 w339 w348 w366 w372]
          tunnel: w138 -> [w156 w177 w213 w230 w238 w251 w262 w268 w286 w308 w326 w342 w351 w369 _]
          tunnel: w137 -> [w155 w176 w211 w228 w236 w249 w261 w266 w284 w306 w324 w340 w349 w368 w371]
          tunnel: [w155 w176 w211 w228 w236 w249 w261 w266 w284 w306 w324 w340 w349 w368 w371] -> w136
          tunnel: w135 -> [w152 w175 _ w214 w234 w243 w259 w264 w282 w290 w323 w327 w346 w367 w370]
          tunnel: [w152 w175 w206 w214 w234 w243 w259 w264 w282 w290 w323 w327 w346 w367 w370] -> w134
          event "btnCalcPFI": Value Change {
            n74 = event-data() -> ()  [unwired: 1 in, 1 out]
            n75 = call <vilib>:"Set Busy.vi"("error in (no error)"=w154) -> ("error out"=w148:errorcluster)  [unwired: 9 in, 1 out]
            n76 = property on="rdoTest Type" class="RadioBtnsControl (strict)"(error in=w148) -> (error out=w147:errorcluster, "Value"=w146:enum32{"rFull", "rTemp"})  [unwired: 1 in, 1 out]
            n77 = case shown="\"rFull\", Default" w146 {
              tunnel: w157 -> [w164 w167]
              tunnel: w155 -> [w163 w168]
              tunnel: w147 -> [w162 w170]
              tunnel: [w160 w169] -> w151
              frame "rFull", Default {
                n78 = call "fgRptEna.vi"("eRptType"=T11."Set PFI" ("Enum")) -> ()  [unwired: 10 in, 1 out]
                n79 = call "CalcSummaryUncertainties.vi"("error in (no error)"=w162, "Limits"=w163, "Uncertainties"=w164) -> ("error out"=w160:errorcluster, "PFI"=→"PFI":string[][][])  [unwired: 7 in]
              }
              frame "rTemp" {
                n80 = call "CalcSummaryUncertainties_TempTest.vi"("error in (no error)"=w170, "Limits"=w168, "Uncertainties"=w167) -> ("error out"=w169:errorcluster, "PFI"=→"Temp Test PFI":string[][][])  [unwired: 7 in]
                n81 = call "fgRptEna.vi"("eRptType"=T11."Set Temp" ("Enum")) -> ()  [unwired: 10 in, 1 out]
              }
            }
            n82 = property on="Tab Control" class="TabCtl (strict)"(error in=w151, "Value"=T2."S.S. & Dyn" ("Tab Control")) -> (error out=w150:errorcluster)  [unwired: 1 in, 1 out]
            n83 = call <vilib>:"Unset Busy.vi"("error in (no error)"=w150) -> ("error out"=w153:errorcluster)  [unwired: 10 in]
          }
          event Value Change {
            n84 = event-data() -> ("NewVal"=w173:T1)  [unwired: 1 in]
            n85 = case shown="\"rFull\", Default" w173 {
              tunnel: w172 -> [w182 w184]
              tunnel: [w180 w186] -> w171
              frame "rFull", Default {
                n86 = property on="btnCalcRT" class="Bool"(error in=w182, "DisabledEnum"=T7."Enabled" ("Disabled")) -> (error out=w180:errorcluster)  [unwired: 1 in, 1 out]
                n87 = property on="full_temp_PFI" class="TabCtl (strict)"("Value"=enum32{"full", "temp"}."full" ("full_temp_PFI")) -> ()  [unwired: 2 in, 2 out]
              }
              frame "rTemp" {
                n88 = property on="full_temp_PFI" class="TabCtl (strict)"(error in=w184, "Value"=enum32{"full", "temp"}."temp" ("full_temp_PFI")) -> (error out=w183:errorcluster)  [unwired: 1 in, 1 out]
                n89 = property on="btnCalcRT" class="Bool"(error in=w184, "DisabledEnum"=T7."Disabled and Grayed Out" ("Disabled")) -> (error out=w187:errorcluster)  [unwired: 1 in, 1 out]
                n90 = Merge Errors(w183, w187) -> (w186:errorcluster)
              }
            }
          }
          event "btnCalcRT": Value Change {
            n91 = event-data() -> ()  [unwired: 1 in, 1 out]
            n92 = call <vilib>:"Set Busy.vi"("error in (no error)"=w209) -> ("error out"=w208:errorcluster)  [unwired: 9 in, 1 out]
            n93 = call "fgRptEna.vi"("eRptType"=T11."Set Step" ("Enum")) -> ()  [unwired: 10 in, 1 out]
            n94 = call "CalcStepUncertainty.vi"("error in (no error)"=w208, "Limits"=w211, "Uncertainties"=w212) -> ("error out"=w190:errorcluster, "clDlyTime"=w198:T12, "clOvrUndr"=w201:T13, "Step Error"=w210:dbl[][][][][], "clRespTime"=w205:T14, "StepData"=w206:dbl[][][][][])  [unwired: 3 in]
            n95 = Unbundle By Name(w205) -> ("RT Range"=→"RTRange":dbl[][][][][], "RT Uncert"=→"RTUncert":dbl[][][][][], "RT_PFI"=→"RTPFI":string[][][])
            n96 = Unbundle By Name(w198) -> ("DlyTimeRng"=→"DlyTimeRng":dbl[][][][][], "DlyTimePFI"=→"DlyTimePFI":string[][][])
            n97 = Unbundle By Name(w201) -> ("OvrUndr"=→"OvrUndr":dbl[][][][][], "OvrUndrPFI"=→"OvrUndrPFI":string[][][][][])
            n98 = property on="ctlPlot" class="Clust (strict)"(error in=w190, "Val(Sgnl)"=T6 {"Channel"=enum."VA", "Parameter"=enum."TVE"} ("Value (Signaling)")) -> (error out=w194:errorcluster)  [unwired: 1 in, 1 out]
            n99 = property on="Tab Control" class="TabCtl (strict)"(error in=w190, "Value"=T2."Step Plot" ("Tab Control")) -> (error out=w191:errorcluster)  [unwired: 1 in, 1 out]
            n100 = Merge Errors(w194, w191) -> (w192:errorcluster)
            n101 = call <vilib>:"Unset Busy.vi"("error in (no error)"=w192) -> ("error out"=w207:errorcluster)  [unwired: 10 in]
          }
          event "ePlotDir", "ePlotType": Value Change {
            w222 = u32 0 ("element")
            n102 = event-data() -> ()  [unwired: 1 in, 1 out]
            n103 = To Unsigned Long Integer(number="ePlotType") -> (unsigned 32bit integer=w224:u32)
            n104 = To Unsigned Long Integer(number="ePlotDir") -> (unsigned 32bit integer=w223:u32)
            n105 = To Unsigned Long Integer(number="ePlotPage") -> (unsigned 32bit integer=w225:u32)
            n106 = Build Array(w225, w224, w223, w222, w222) -> (w219:u32[])
            n107 = call "PlotStep.vi"("StepPlotData"=w214, "index"=w219, "ctlPlot"="ctlPlot", "StepTVEData"=w221) -> ("StepPlot"=→"StepPlot":cluster{"Array":dbl[], "Array":dbl[]}, "StepTVE"=→"Step TVE":cluster{"Array":dbl[], "Array":dbl[]})  [unwired: 6 in]
          }
          event Value Change {
            w240 = u32 0 ("element")
            n108 = event-data() -> ()  [unwired: 1 in, 1 out]
            n109 = To Unsigned Long Integer(number="Limit Page") -> (unsigned 32bit integer=w241:u32)
            n110 = Build Array(w241, w240, w240) -> (w231:u32[])
            n111 = property on="StepLimits" class="Arr (strict)"(error in=w233, "Index Values"=w231) -> (error out=w232:errorcluster)  [unwired: 1 in, 1 out]
            n112 = property on="Limits" class="Arr (strict)"(error in=w232, "Index Values"=w231) -> (error out=w239:errorcluster)  [unwired: 1 in, 1 out]
          }
          event Value Change {
            w245 = 0
            n113 = event-data() -> ()  [unwired: 1 in, 1 out]
            n114 = Build Array("TUR Page", w245, w245) -> (w244:i32[])
            n115 = property on="TUR" class="Arr (strict)"(error in=w247, "Index Values"=w244) -> (error out=w252:errorcluster)  [unwired: 1 in, 1 out]
          }
          event "UncertPage": Value Change {
            n116 = event-data() -> ()  [unwired: 1 in, 1 out]
            n117 = To Unsigned Long Integer(number="UncertPage") -> (unsigned 32bit integer=w257:u32)
            n118 = Index Array(array=w258, index (dim 0)=w257) -> (element=w256:dbl[][])  [unwired: 2 in]
            n119 = call "Uncert Table Layout.vi"("Uncert In"=w256) -> ("Uncert Table"=w253:string[][])  [unwired: 10 in]
            n120 = property on="Uncert Table" class="Tbl (strict)"(error in=w255, "Value"=w253) -> (error out=w254:errorcluster)  [unwired: 1 in, 1 out]
          }
          event Value Change {
            w270 = 0
            n121 = event-data() -> ()  [unwired: 1 in, 1 out]
            n122 = Build Array("PFI Page", w270, w270) -> (w269:i32[])
            n123 = property on="PFI" class="Arr (strict)"(error in=w272, "Index Values"=w269) -> (error out=w273:errorcluster)  [unwired: 1 in, 1 out]
          }
          event "TempFreq": Value Change {
            w287 = 0
            n124 = event-data() -> ()  [unwired: 1 in, 1 out]
            n125 = control-ref of="full_temp_PFI"() -> (w278:refnum<vi>)
            n126 = Build Array("TempFreq", w287, w287) -> (w280:i32[])
            n127 = case shown="\"60 Hz\"" "TempFreq" {
              tunnel: [1 0] -> w274
              frame "50 Hz", Default {
              }
              frame "60 Hz" {
              }
            }
            n128 = property on="Temp Test PFI" class="Arr (strict)"(error in=w279, "Index Values"=w280) -> (error out=w281:errorcluster)  [unwired: 1 in, 1 out]
            n129 = call "LblTgl.vi"("TabControl in"=w278, "Numeric"=w274) -> ("error out"=w276:errorcluster)  [unwired: 17 in]
            n130 = Merge Errors(w276, w281) -> (w277:errorcluster)
          }
          event Value Change {
            w294 = u32 0 ("element")
            w300 = u32 0 ("element")
            n131 = event-data() -> ()  [unwired: 1 in, 1 out]
            n132 = To Unsigned Long Integer(number="eRTType") -> (unsigned 32bit integer=w302:u32)
            n133 = To Unsigned Long Integer(number="eRTDir") -> (unsigned 32bit integer=w301:u32)
            n134 = To Unsigned Long Integer(number="eRTPage") -> (unsigned 32bit integer=w295:u32)
            n135 = Build Array(w295, w294, w294) -> (w291:u32[])
            n136 = property on="RTPFI" class="Arr (strict)"(error in=w293, "Index Values"=w291) -> (error out=w292:errorcluster)  [unwired: 1 in, 1 out]
            n137 = Build Array(w295, w302, w301, w300, w300) -> (w299:u32[])
            n138 = property on="RTRange" class="Arr (strict)"(error in=w292, "Index Values"=w299) -> (error out=w303:errorcluster)  [unwired: 1 in, 1 out]
            n139 = property on="RTUncert" class="Arr (strict)"(error in=w303, "Index Values"=w299) -> (error out=w304:errorcluster)  [unwired: 1 in, 1 out]
          }
          event Value Change {
            w317 = u32 0 ("element")
            w319 = u32 0 ("element")
            n140 = event-data() -> ()  [unwired: 1 in, 1 out]
            n141 = To Unsigned Long Integer(number="eDTType") -> (unsigned 32bit integer=w321:u32)
            n142 = To Unsigned Long Integer(number="eDTDir") -> (unsigned 32bit integer=w320:u32)
            n143 = To Unsigned Long Integer(number="eDTPage") -> (unsigned 32bit integer=w318:u32)
            n144 = Build Array(w318, w317, w317) -> (w309:u32[])
            n145 = Build Array(w318, w321, w320, w319, w319) -> (w312:u32[])
            n146 = property on="DlyTimePFI" class="Arr (strict)"(error in=w310, "Index Values"=w309) -> (error out=w311:errorcluster)  [unwired: 1 in, 1 out]
            n147 = property on="DlyTimeRng" class="Arr (strict)"(error in=w311, "Index Values"=w312) -> (error out=w313:errorcluster)  [unwired: 1 in, 1 out]
          }
          event Value Change {
            w329 = 0
            n148 = event-data() -> ()  [unwired: 1 in, 1 out]
            n149 = To Unsigned Long Integer(number="eOvrUndrPage") -> (unsigned 32bit integer=w332:u32)
            n150 = To Unsigned Long Integer(number="eOvrDir") -> (unsigned 32bit integer=w330:u32)
            n151 = To Unsigned Long Integer(number="eOvrType") -> (unsigned 32bit integer=w331:u32)
            n152 = Build Array(w332, w331, w330, w329, w329) -> (w328:u32[])
            n153 = property on="OvrUndrPFI" class="Arr (strict)"(error in=w335, "Index Values"=w328) -> (error out=w334:errorcluster)  [unwired: 1 in, 1 out]
            n154 = property on="OvrUndr" class="Arr (strict)"(error in=w334, "Index Values"=w328) -> (error out=w333:errorcluster)  [unwired: 1 in, 1 out]
          }
          event "btnSave": Value Change {
            n155 = event-data() -> ()  [unwired: 1 in, 1 out]
            n156 = property on="rdoTest Type" class="RadioBtnsControl (strict)"(error in=w344) -> (error out=w343:errorcluster, "Value"=w345:enum32{"rFull", "rTemp"})  [unwired: 1 in, 1 out]
            n157 = case shown="\"rTemp\"" w345 {
              tunnel: w343 -> [w357 w360]
              tunnel: [w356 w359] -> w347
              frame "rFull", Default {
                n158 = property on="RTPFI" class="Arr (strict)"() -> ("Value"=w355:string[][][])  [unwired: 2 in, 2 out]
                n159 = property on="PFI" class="Arr (strict)"() -> ("Value"=w354:string[][][])  [unwired: 2 in, 2 out]
                n160 = property on="OvrUndrPFI" class="Arr (strict)"() -> ("Value"=w353:string[][][][][])  [unwired: 2 in, 2 out]
                n161 = property on="DlyTimePFI" class="Arr (strict)"() -> ("Value"=w352:string[][][])  [unwired: 2 in, 2 out]
                n162 = call "WritePFIReport.vi"("RT PFI"=w355, "error in (no error)"=w357, "DT PFI"=w352, "Ovrshoot PFI"=w353, "PFI"=w354) -> ("error out"=w356:errorcluster)  [unwired: 6 in]
              }
              frame "rTemp" {
                n163 = property on="Temp Test PFI" class="Arr (strict)"() -> ("Value"=w358:string[][][])  [unwired: 2 in, 2 out]
                n164 = call "WritePFIReport_TempTest.vi"("error in (no error)"=w360, "Temp PFI"=w358) -> ("error in (no error) 2"=w359:errorcluster)  [unwired: 9 in]
              }
            }
          }
          event "btnSaveTUR": Value Change {
            n165 = event-data() -> ()  [unwired: 1 in, 1 out]
            n166 = property on="TUR" class="Arr (strict)"(error in=w364) -> (error out=w363:errorcluster, "Value"=w362:dbl[][][])  [unwired: 1 in, 1 out]
            n167 = call "WriteUncTURReport.vi"("error in (no error)"=w363, "TUR"=w362, "UNC"=w361) -> ("error out"=w365:errorcluster)  [unwired: 8 in]
          }
          event "DONE": Value Change {
            n168 = event-data() -> ()  [unwired: 1 in, 1 out]
          }
        }
        n169 = property on="rdoTest Type" class="RadioBtnsControl (strict)"(error in=w131) -> (error out=w130:errorcluster, "Value"=w129:enum32{"rFull", "rTemp"})  [unwired: 1 in, 1 out]
        n170 = call "fgRptEna.vi"("eRptType"=T11."get" ("Enum"), "rdoTest Type"=w129) -> ("ENA"=w128:T7)  [unwired: 9 in]
        n171 = property on="btnSave" class="Bool"(error in=w130, "DisabledEnum"=w128) -> (error out=w133:errorcluster)  [unwired: 1 in, 1 out]
      }
      frame "exit" {
      }
    }
    "Uncertainties" <- w95
    n172 = call <vilib>:"Clear Errors.vi"("error in (no error)"=w89, "specific error code to clear (0: all)"=5002 ("error code (0)")) -> ("error out"=w90:errorcluster)  [unwired: 4 in, 1 out]
    "error out" <- w90
  }
  n173 = control-ref of="This VI"() -> (w1:refnum<vi>)
  n174 = invoke class="VI" method="FP.Close"(reference=w1, error in=w18) -> ()  [unwired: 1 in, 3 out]
